vi "Report.New.vi"() -> (1 "TestTime":T1, 3 "TestRecord":T2)   [LabVIEW 2012, in "Lib_UEL.ATE.lvlib" / "Lib_Report.lvlib"]
uses:
  Lib_Report.lvlib
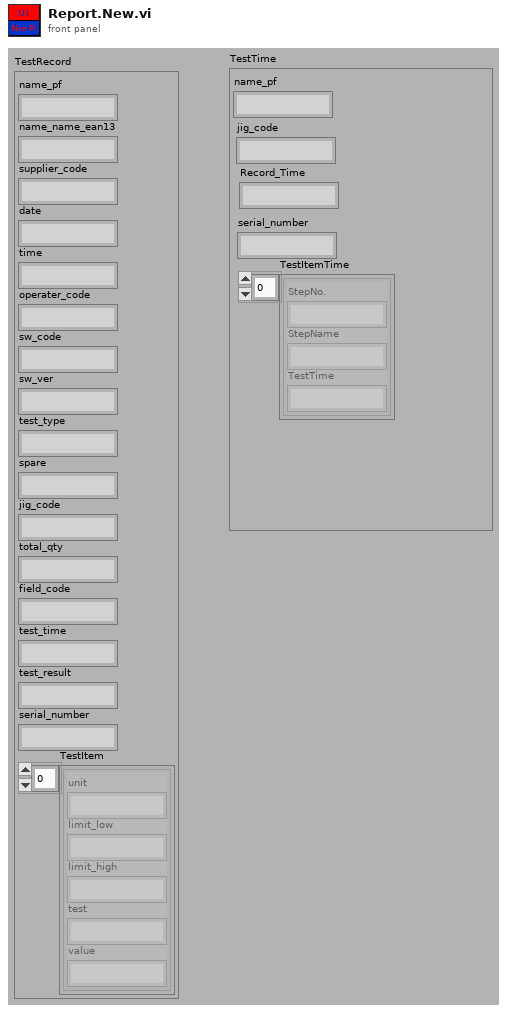
[diagram p1: front panel]
types:
  T1 = cluster{"name_pf":string, "jig_code":string, "Record_Time":string, "serial_number":string, "TestItemTime":cluster{"StepNo.":string, "StepName":string, "TestTime":string}[]}
  T2 = cluster{"name_pf":string, "name_name_ean13":string, "supplier_code":string, "date":string, "time":string, "operater_code":string, "sw_code":string, "sw_ver":string, "test_type":string, "spare":string, "jig_code":string, "total_qty":string, "field_code":string, "test_time":string, "test_result":string, "serial_number":string, "TestItem":cluster{"unit":string, "limit_low":string, "limit_high":string, "test":string, "value":string}[]}
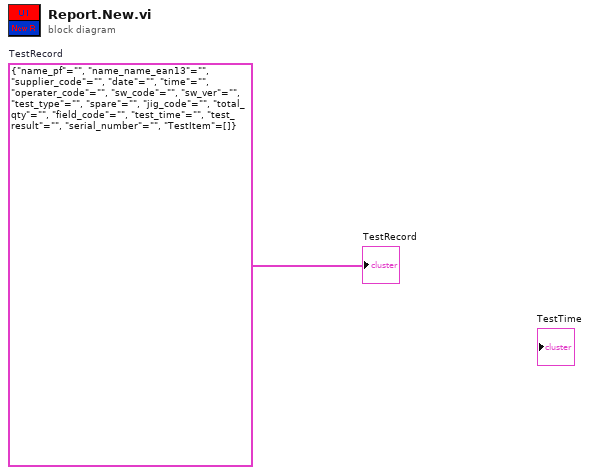
[diagram p0: block diagram]
diagram:
  w1 = T2 {"name_pf"="", "name_name_ean13"="", "supplier_code"="", "date"="", "time"="", "operater_code"="", "sw_code"="", "sw_ver"="", "test_type"="", "spare"="", "jig_code"="", "total_qty"="", "field_code"="", "test_time"="", "test_result"="", "serial_number"="", "TestItem"=[]}  # TestRecord
  "TestRecord" <- w1
